vi "check_IPC_channel.vi"(8 "error in (no error)":errorcluster, 10 "ParamIn":u8, 11 "app_data in":T1) -> (0 "error out":errorcluster, 2 "Telemetry":sgl[](array[numeric]), 3 "app_data out":T1)   [LabVIEW 2017]
uses:
  controls/app_data.ctl
  controls/instruments.ctl
  Unicorn Labview Library/Control/unicorn_Param.ctl
  Unicorn Labview Library/Control/unicorn_conn.ctl
  Unicorn Labview Library/Control/unicorn_JSON.ctl
  Unicorn Labview Library/Control/unicorn_ParamInt.ctl
  Unicorn Labview Library/Control/unicorn_Telemetry.ctl
  Unicorn Labview Library/Control/unicorn_Table.ctl
  Unicorn Labview Library/Control/unicorn_ParamFloat.ctl
  Unicorn Labview Library/Unicorn Library.lvlib
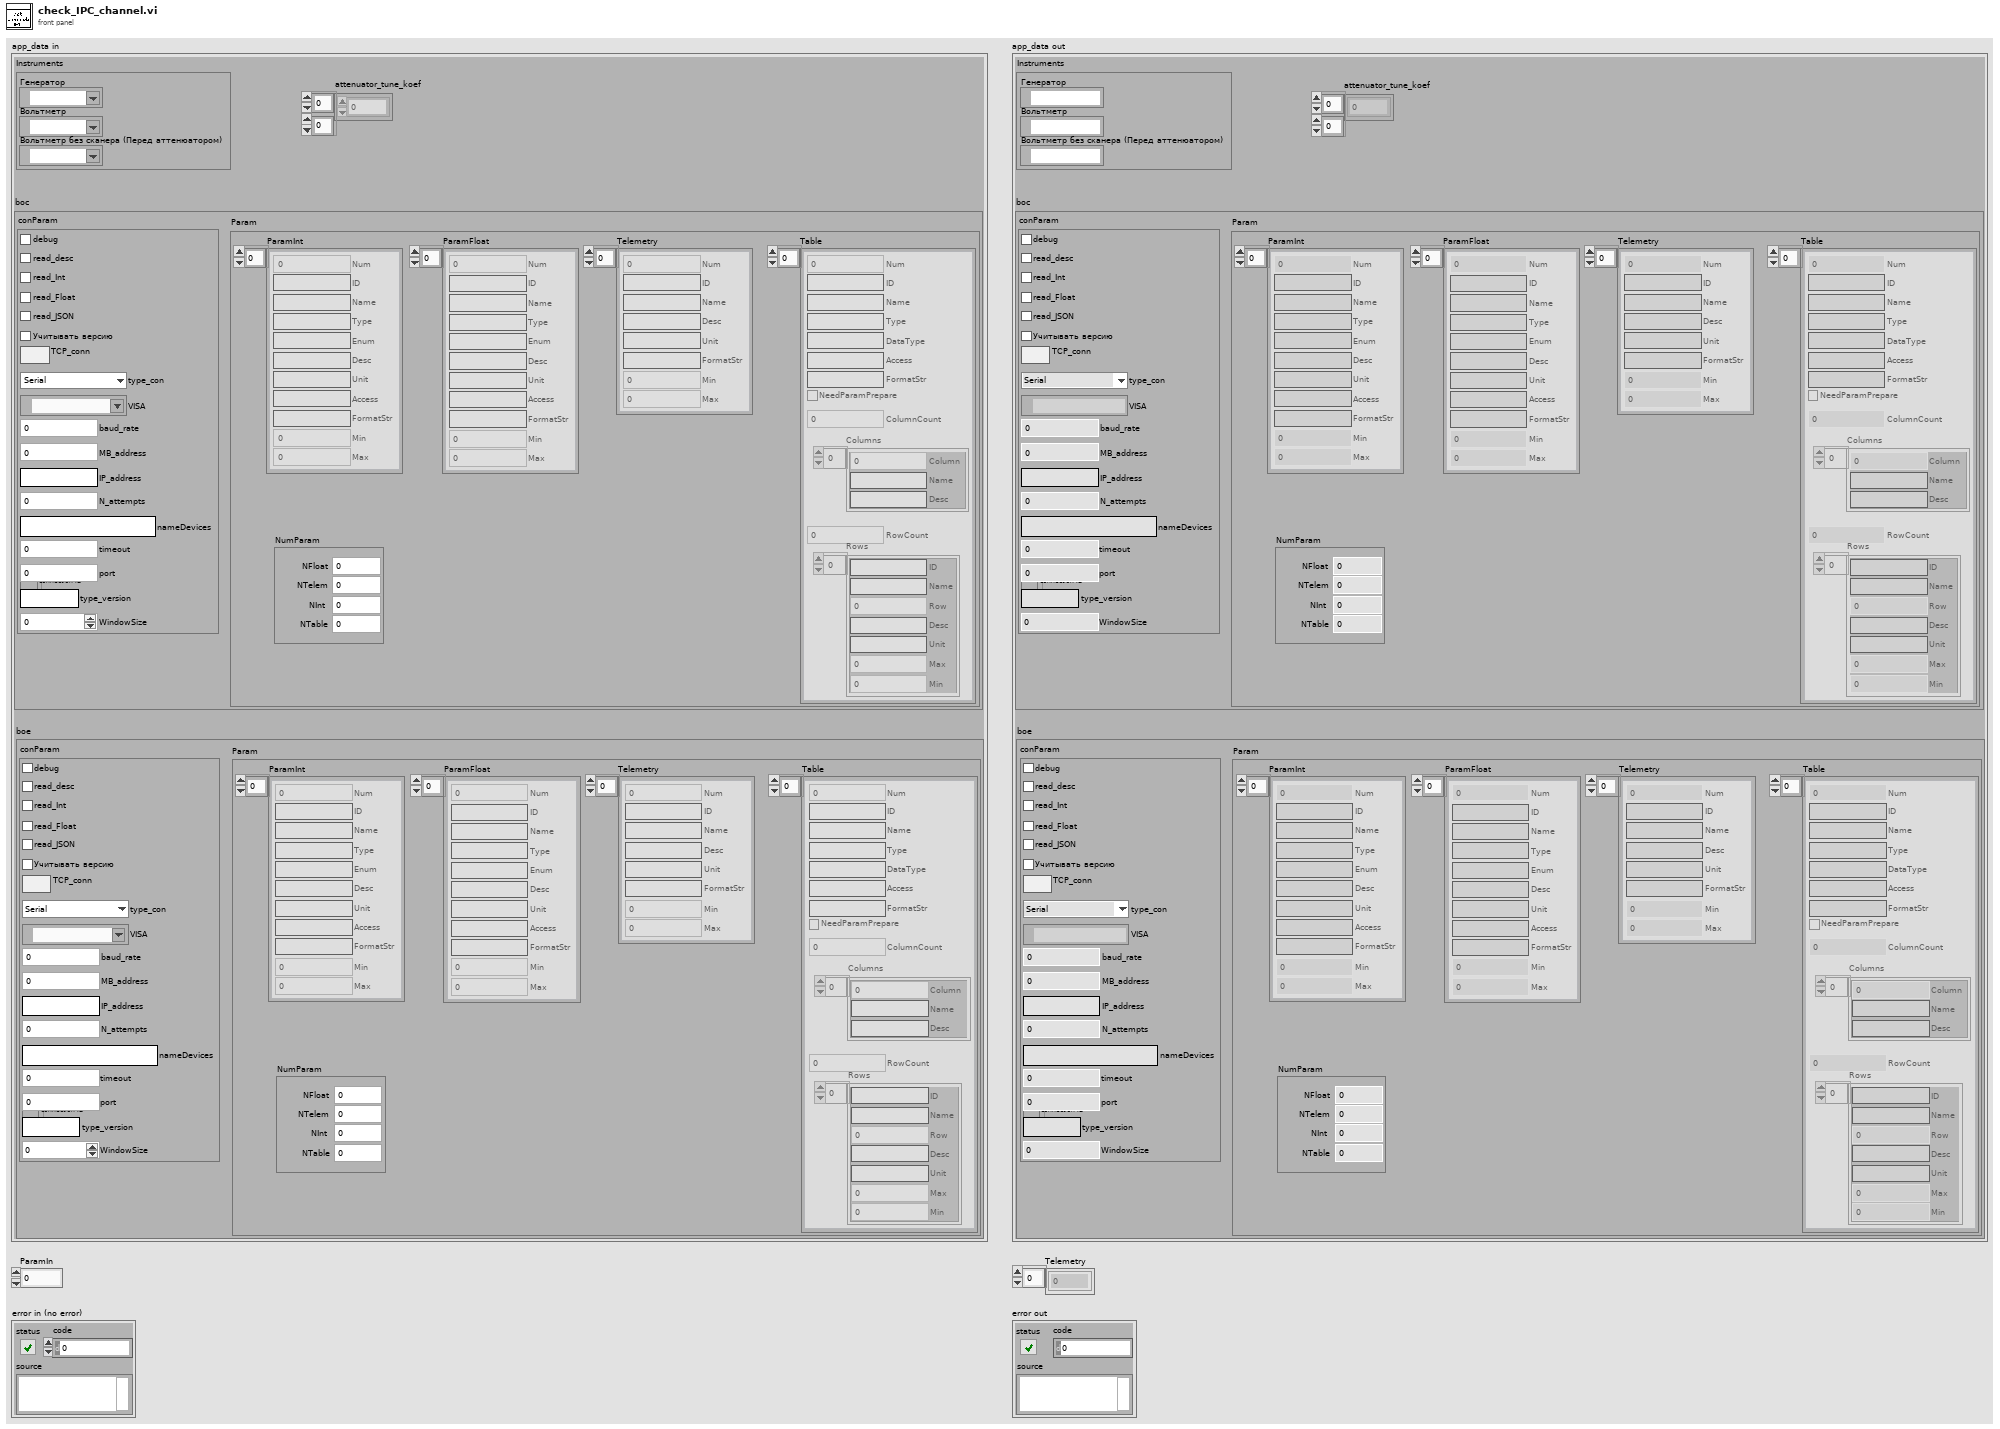
[diagram p1: front panel]
types:
  T1 = typedef "app_data.ctl" = cluster{"Instruments":T2, "boc":T3, "boe":T3, "attenuator_tune_koef":dbl[][]}
  T2 = typedef "instruments.ctl" = cluster{"generator":refnum<visa-resource-name>, "voltment_with_scaner":refnum<visa-resource-name>, "voltment_without_scaner":refnum<visa-resource-name>}
  T3 = typedef "Unicorn Library.lvlib/unicorn_Param.ctl" = cluster{"conParam":T4, "Param":T5}
  T4 = typedef "Unicorn Library.lvlib/unicorn_conn.ctl" = cluster{"ReadIntParam":bool, "ReadDescrParam":bool, "ReadFloatParam":bool, "debug":bool, "ReadJSON":bool, "IP_address":string, "N_attempts":i32, "type_con":enum16{"Serial", "TCP"}, "MB_address":i32, "VISA":refnum<visa-resource-name>, "connection ID":refnum<k5>, "nameDevices":string, "timeout":i32, "port":u16, "type_version":string, "baud_rate":u32, "VersionControl":bool, "TCP_conn":bool, "WindowSize":i32}
  T5 = typedef "Unicorn Library.lvlib/unicorn_JSON.ctl" = cluster{"NumParam":cluster{"NTelem":i32, "NInt":i32, "NFloat":i32, "NTable":i32}, "ParamInt":T6, "Telemetry":T7, "Table":T8, "ParamFloat":T9}
  T6 = typedef "Unicorn Library.lvlib/unicorn_ParamInt.ctl" = cluster{"ID":string, "Num":i32, "Name":string, "Type":string, "Enum":string, "Desc":string, "Unit":string, "Access":string, "FormatStr":string, "Min":i32, "Max":i32}[]
  T7 = typedef "Unicorn Library.lvlib/unicorn_Telemetry.ctl" = cluster{"ID":string, "Num":i32, "Name":string, "Desc":string, "Unit":string, "FormatStr":string, "Min":i32, "Max":i32}[]
  T8 = typedef "Unicorn Library.lvlib/unicorn_Table.ctl" = cluster{"Num":i32, "Access":string, "ColumnCount":i32, "NeedParamPrepare":bool, "Columns":cluster{"Column":i32, "Desc":string, "Name":string}[], "DataType":string, "FormatStr":string, "ID":string, "Name":string, "RowCount":i32, "Rows":cluster{"Desc":string, "ID":string, "Max":i32, "Min":i32, "Name":string, "Row":i32, "Unit":string}[], "Type":string}[]
  T9 = typedef "Unicorn Library.lvlib/unicorn_ParamFloat.ctl" = cluster{"ID":string, "Num":i32, "Name":string, "Type":string, "Enum":string, "Desc":string, "Unit":string, "Access":string, "FormatStr":string, "Min":i32, "Max":i32}[]
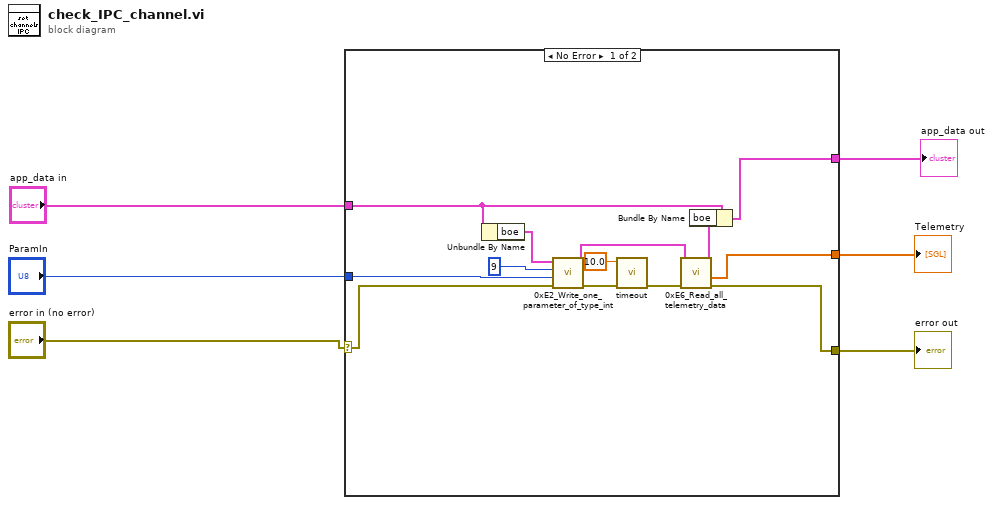
[diagram p0: block diagram]
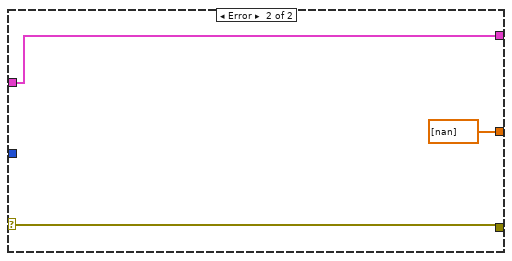
[diagram p2: hidden frame]
diagram:
  n1 = case shown="No Error" "error in (no error)" {
    selector: "error in (no error)" -> [w7 w22]
    tunnel: [w19 sgl[] [nan] ("Telemetry")] -> w6
    tunnel: [w18 w22] -> w5
    tunnel: [w17 w21] -> w4
    tunnel: "app_data in" -> [w15 w21]
    tunnel: "ParamIn" -> [w11 _]
    frame No Error {
      n2 = Unbundle By Name(w15) -> ("boe"=w13:T3)
      n3 = call "0xE2_Write_one_parameter_of_type_int.vi"("error in"=w7, "ParamIn"=w11, "NumParamIn"=9, "paramUnicorn 2"=w13) -> ("error out"=w10:errorcluster, "paramUnicornOut"=w14:T3)  [unwired: 4 in, 2 out]
      n4 = call "timeout.vi"("error in (no error)"=w10, "seconds to wait"=10.0) -> ("error IO"=w9:errorcluster)  [unwired: 9 in]
      n5 = call "0xE6_Read_all_telemetry_data.vi"("error in"=w9, "paramUnicorn"=w14) -> ("error out"=w18:errorcluster, "Telemetry"=w19:sgl[], "paramUnicorn 2"=w16:T3)  [unwired: 5 in, 1 out]
      n6 = Bundle By Name(cluster=w15, "boe"=w16) -> (w17:T1)
    }
    frame Error {
    }
  }
  "Telemetry" <- w6
  "error out" <- w5
  "app_data out" <- w4
